vi "Full Build Assert.vi"(8 "error in (no error)":errorcluster, 10 "GObj Refnum":refnum<vi>, 11 "VI in":refnum<vi>) -> (0 "error out":errorcluster)   [LabVIEW 2018]
doc: "Full build process from start to finish for a single assert"
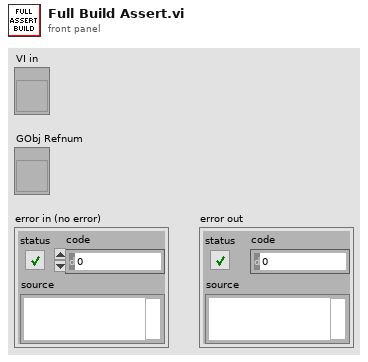
[diagram p1: front panel]
types:
  T1 = typedef "NI_Data Type.lvlib/Data Type.ctl" = enum8{"Invalid Type", "Void", "I8", "I16", "I32", "I64", "U8", "U16", "U32", "U64", "Single Float", "Double Float", "Extended Float", "Single Complex", "Double Complex", "Extended Complex", "Enum U8", "Enum U16", "Enum U32", "Enum U64", "Single Float With Unit", "Double Float With Unit", "Extended Float With Unit", "Single Complex with Unit", "Double Complex with Unit", "Extended Complex with Unit", "Boolean", "String", "Path", "Picture", "Tag", "Array", "Cluster", "Variant", "LV Variant", "Waveform", "Timestamp", "Digital Waveform", "Digital Data", "ExpressData", "Refnum", "External Data", "VI", "Poly VI", "LabVIEW Class Instance", "Fixed Point"}
  T2 = typedef "Assert Add Configuration.ctl" = cluster{"Include Evaluation String Comment":bool, "Inline or Forked":T3, "Eval String":string}
  T3 = typedef "Inline or Forked.ctl" = enum32{"Inline", "Forked"}
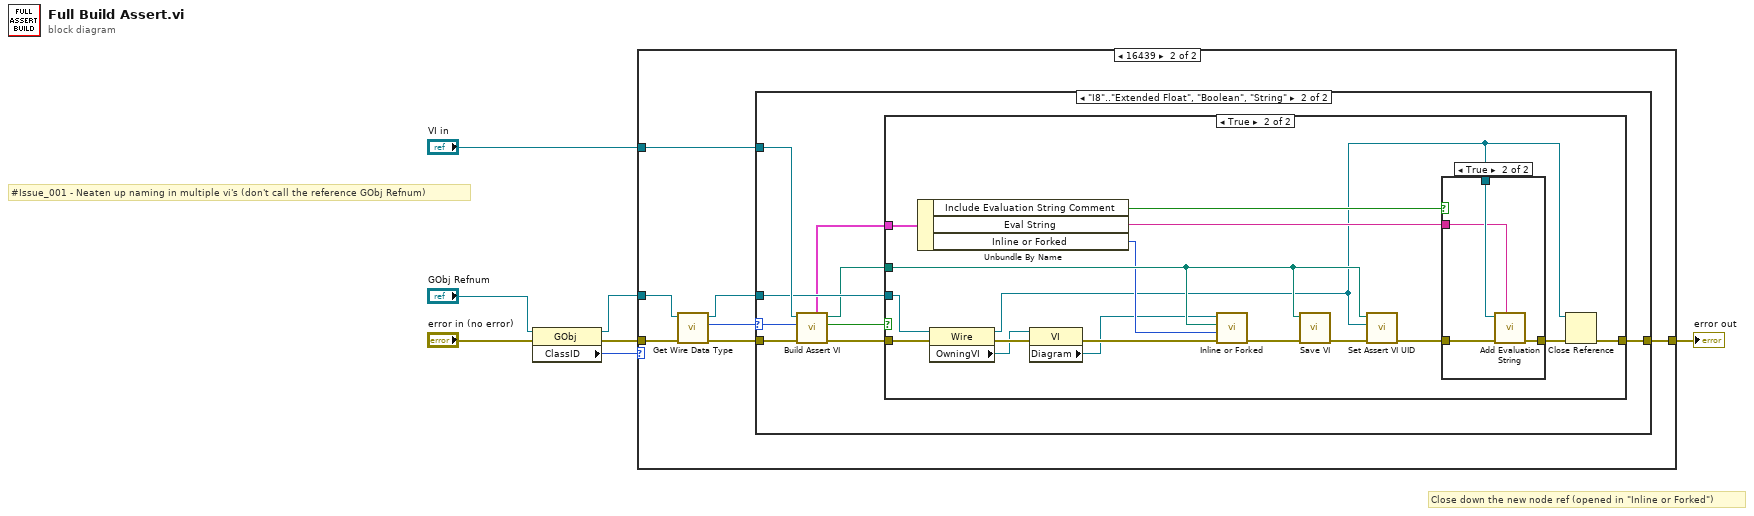
[diagram p0: block diagram]
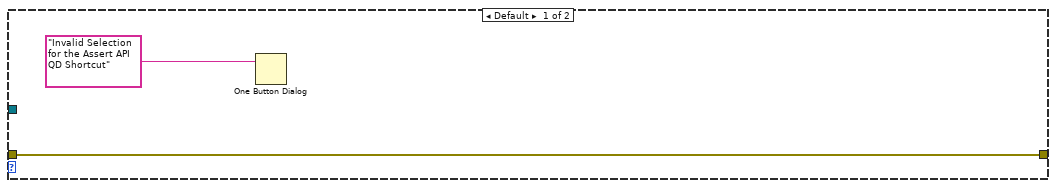
[diagram p2: hidden frame]
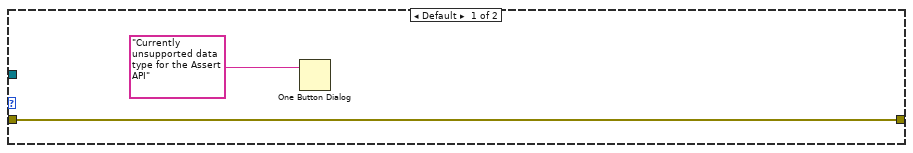
[diagram p3: hidden frame]
diagram:
  # "#Issue_001 - Neaten up naming in multiple vi's (don't call the reference GObj Refnum)"
  # "Close down the new node ref (opened in \"Inline or Forked\")"
  n1 = property class="GObj"(reference="GObj Refnum", error in="error in (no error)") -> (reference out=w5:refnum<vi>, error out=w4:errorcluster, "ClassID"=w3:u32)
  n2 = case shown="16439" w3 {
    tunnel: w4 -> [w8 w16]
    tunnel: w5 -> [_ w12]
    tunnel: [w8 w14] -> w6
    tunnel: "VI in" -> [_ w13]
    frame Default {
      n3 = One Button Dialog(message="Invalid Selection for the Assert API QD Shortcut") -> ()  [unwired: 1 in, 1 out]
    }
    frame 16439 {
      n4 = call "Get Wire Data Type.vi"("error in (no error)"=w16, "Wire ref in"=w12) -> ("error out"=w15:errorcluster, "Type"=w10:T1, "Wire ref out"=w11:refnum<vi>)  [unwired: 7 in]
      n5 = case shown="\"I8\"..\"Extended Float\", \"Boolean\", \"String\"" w10 {
        selector: w10 -> [_ w25]
        tunnel: w15 -> [w18 w27]
        tunnel: [w18 w23] -> w14
        tunnel: w13 -> [_ w26]
        tunnel: w11 -> [_ w22]
        frame Default {
          n6 = One Button Dialog(message="Currently unsupported data type for the Assert API") -> ()  [unwired: 1 in, 1 out]
        }
        frame "I8".."Extended Float", "Boolean", "String" {
          n7 = call "Build Assert VI.vi"("error in (no error)"=w27, "Type"=w25, "VI Refnum"=w26) -> ("error out"=w24:errorcluster, "Add Object"=w20:bool, "appended path"=w21:path, "Assert Add Configuration"=w19:T2)  [unwired: 5 in]
          n8 = case shown="True" w20 {
            tunnel: w24 -> [w28 w34]
            tunnel: [w28 w36] -> w23
            tunnel: w22 -> [_ w35]
            tunnel: w21 -> [_ w42]
            tunnel: w19 -> [_ w40]
            frame False {
            }
            frame True {
              n9 = Unbundle By Name(w40) -> ("Include Evaluation String Comment"=w39:bool, "Eval String"=w38:string, "Inline or Forked"=w37:T3)
              n10 = property class="Wire"(reference=w35, error in=w34) -> (reference out=w29:refnum<vi>, error out=w33:errorcluster, "OwningVI"=w31:refnum<vi>)
              n11 = property class="VI"(reference=w31, error in=w33) -> (error out=w32:errorcluster, "Diagram"=w30:refnum<vi>)  [unwired: 1 out]
              n12 = call "Inline or Forked.vi"("error in (no error)"=w32, "Inline or Forked"=w37, "Assert VI Path"=w42, "Diagram in"=w30) -> ("error out"=w45:errorcluster)  [unwired: 7 in]
              n13 = call "Save VI.vi"("error in (no error)"=w45, "Assert VI Path"=w42) -> ("error out"=w44:errorcluster)  [unwired: 9 in]
              n14 = call "Set Assert VI UID.vi"("error in (no error)"=w44, "GObj Refnum"=w29, "Assert VI Path"=w42) -> ("error out"=w43:errorcluster)  [unwired: 8 in]
              n15 = case shown="True" w39 {
                tunnel: w43 -> [w46 w50]
                tunnel: [w46 w49] -> w41
                tunnel: w29 -> [_ w48]
                tunnel: w38 -> [_ w47]
                frame False {
                }
                frame True {
                  n16 = call "Add Evaluation String.vi"("Evaluation String"=w47, "error in (no error)"=w50, "GObj Refnum"=w48) -> ("error out"=w49:errorcluster)  [unwired: 8 in]
                }
              }
              n17 = Close Reference(reference=w29, error in (no error)=w41) -> (error out=w36:errorcluster)
            }
          }
        }
      }
    }
  }
  "error out" <- w6
